vi "DN4_Counter_SetDelayCount_Ex.vi"(3 "error in (no error)":errorcluster, 4 "delay count":i32[](array[numeric]), 5 "Task ID":u32) -> (0 "error out":errorcluster, 2 "Task ID":u32)   [LabVIEW 2009]
uses:
  Windows/System32/AdvLvDaq.dll
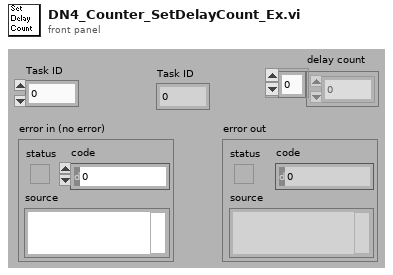
[diagram p1: front panel]
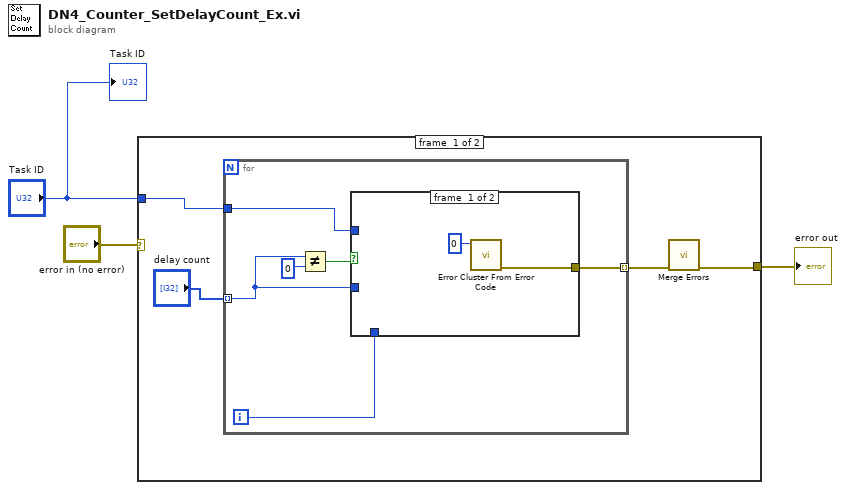
[diagram p0: block diagram]
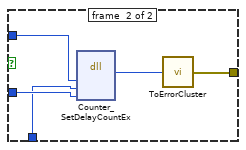
[diagram p2: hidden frame]
diagram:
  n1 = case shown="No Error" "error in (no error)" {
    selector: "error in (no error)" -> [_ w21]
    tunnel: [w4 w21] -> w1
    tunnel: "Task ID" -> [w7 _]
    frame #0 {
      n2 = for {
        tunnel: w7 -> [w11]
        tunnel: "delay count" -> [w10] mode=indexing
        tunnel: [w8] -> w5 mode=indexing
        i -> [w9]
        n3 = Not Equal?(x=w10, y=0) -> (x != y?=w12:bool)
        n4 = case shown="True" w12 {
          tunnel: w11 -> [_ w20]
          tunnel: w10 -> [_ w19]
          tunnel: w9 -> [_ w18]
          tunnel: [w14 w16] -> w8
          frame #0 {
            n5 = call <vilib>:"Error Cluster From Error Code.vi"("error code (0)"=0) -> ("error out"=w14:errorcluster)  [unwired: 2 in, 6 out]
          }
          frame #1 {
            n6 = dll-call lib="C:/Windows/System32/AdvLvDaq.dll" fn="Counter_SetDelayCountEx"("taskId"=w20, "channelIndex"=w18, "delayCount"=w19) -> ("return type"=w17:i32)  [unwired: 6 in, 2 out]
            n7 = call <userlib>:"ToErrorCluster.vi"("error code"=w17) -> ("error out"=w16:errorcluster)
          }
        }
      }
      n8 = call <vilib>:"Merge Errors.vi"("error array in"=w5) -> ("error out"=w4:errorcluster)  [unwired: 3 in, 3 out]
    }
    frame #1 {
    }
  }
  "error out" <- w1
  "Task ID" <- "Task ID"
